vi "findcurrentpointinpath.vi"(9 "xyhc_in":T3={"idx"=1, "x"=-35.60561147, "y"=-90.69379038, "h"=0.8330275943157105, "x_path"=0.0}, 11 "path_updated":dbl[][](array[numeric])=[[-35.60561147, 14.99557688, 95.95172474, 126.8880385, 138.5119907, 141.9032354, 149.677826, 156.712601, 147.13884, 113.118729, 91.508095, 52.920765, 32.668774, 17.97715, 6.99827, 8.818146, 6.847322, -18.817772, -52.222027, -83.222168, -125.305626, -155.940872, -175.355911, -209.76741, -251.849823, -281.586182, -300.850311, -306.885162, -303.253143, -295.630493, -278.449524, -230.05719, -162.346695, -115.394356, -97.840988, -93.721558, -107.58947, -152.137314, -214.105331, -237.05452, -248.829102, -256.267426, -252.825378, -236.371918, -181.819519, -112.524597, -63.289055, 37.82652036, 102.9702202, 119.4941108, 132.2853204, 148.4183775, 169.4908835, 199.2599464, 217.8178611, 183.2960532, 161.2291024, 113.8171392, 51.7116428, 18.83330746, -40.94467646, -158.2175499, -304.1845662, -356.4114598, -371.7179639, -364.7774941, -321.8985356, -260.4948464, -177.352901, -134.2672684, -111.7310869, -102.4948394], [-90.69379038, -29.89498053, 67.16989543, 104.5939161, 124.5329647, 150.0144894, 165.817642, 203.642349, 245.81633, 291.834503, 311.325348, 320.550659, 312.945953, 299.664246, 267.743835, 241.541656, 208.411987, 171.587891, 162.666382, 167.037628, 157.857651, 138.040024, 134.616943, 139.73143, 136.464813, 119.024261, 90.540421, 58.270515, 37.237495, 23.16614, 14.112659, 28.614491, 56.741966, 65.419174, 53.848969, 35.074554, 14.354389, -0.839164, -11.569063, -18.164124, -25.487514, -39.475895, -50.265072, -60.782021, -86.859489, -89.836975, -52.336075, 47.42656259, 108.7608178, 124.5858933, 130.5720458, 134.255832, 156.1042719, 192.4121936, 263.2998005, 322.1206095, 338.63727, 360.3326326, 347.82789, 323.5375909, 277.8521386, 199.9919628, 130.779043, 91.89366581, 42.53528347, 5.307577259, -40.68181368, -69.83663356, -108.4425596, -125.3508342, -127.104311, -126.4810207], [0.8330275943157105, 0.8766933449672827, 0.8720608266883365, 0.8763291798774375, 1.4436202967580976, 1.0953588545336055, 1.202427103434421, 1.5675334075735572, 2.0208601993339705, 2.3344985584549347, 2.5217023998013075, 3.2905088869696257, 3.6946919524698116, 4.054443038499433, 4.694786404404647, 4.772122693546571, 4.485709108373563, 3.7189722485083774, 3.0712663600820562, 3.004853495888188, 3.7906498504911594, 3.507009551669314, 3.085443058474223, 3.0170500157627536, 3.451775038358818, 3.8955294400228175, 4.328504950817729, 4.7359268353628785, 5.031782879381744, 5.430482825844485, 6.2394321209923564, 6.667391813220487, 6.668706688268769, 6.092256265390278, 5.302149133586403, 4.529530775971869, 3.8056763953109787, 3.3266811332477855, 3.3420818347587327, 3.5361917912418064, 3.890153235193759, 4.650683955154467, 5.394163658376154, 5.775327394760227, 5.905741446161766, 6.685389788966887, 7.0624439921025415, 7.043797067523052, 7.045860587140642, 6.971258941777836, 6.421503011695177, 6.831190408876256, 7.153447806758524, 7.2239567423466955, 8.010347243061005, 8.72699497983693, 8.805052050684726, 9.26421305386915, 9.962792387892115, 10.087553564759371, 10.0731898733389, 9.920135612491762, 9.858317839615056, 10.401200892986212, 10.975024036193423, 11.393169003772442, 12.079383823703623, 12.12107561568999, 12.126125525723165, 12.365408786334852, 12.620725973569215, 12.60295968190307], [79.02567858668118, 126.39410707077633, 48.55371777691576, 22.760113207585164, 25.705859872710697, 17.609108944674627, 37.82045155891601, 42.14251814120699, 56.23518430452567, 29.023776728286606, 36.76726299353208, 21.15613435953993, 19.4783482417429, 31.97053018080938, 26.16608687203961, 32.95292667454974, 41.65012483034862, 32.85891459850081, 31.230672725830544, 40.43928661324237, 36.384170766299235, 19.35635780443436, 34.64429285631372, 41.35068505459292, 33.64069817064366, 33.54113151797454, 32.18140470915767, 21.112675843186466, 15.753153719369196, 18.122051452076935, 47.711722734111554, 73.31698058485364, 46.769151831896224, 19.43008535281352, 17.893999212117908, 22.89647093243486, 44.44498003577213, 62.884262384730775, 23.802898182097472, 13.685104750022273, 14.97011159822701, 10.556386662163115, 18.53445321010401, 60.34888944373504, 65.51457234068675, 59.98620700193982, 142.04554298999807, 89.47270858101754, 22.879495492192838, 13.682343682882424, 16.486885572353348, 29.369484986199453, 46.9472486010369, 68.21176822330133, 63.47923585020231, 27.521502278658343, 51.19605292655213, 59.307434583487634, 40.68066703288778, 75.23282019763789, 140.49305222582296, 161.32170793131496, 63.730285722300245, 49.46488273601802, 37.07722725836663, 59.00479817964879, 67.90876101874913, 91.66274958229026, 46.182949286236706, 22.432656547398086, 9.256469076869466, 11.245785601783329], [-6.993606016660986e-06, -1.5813147711021443e-07, -4.9412989479727785e-06, 0.0005804982640230092, -0.0005338958044692879, 0.00022896446877936018, 6.310818226633189e-06, 1.4800092263017844e-05, -1.6797654770616777e-05, 5.070149719265486e-05, 0.000115695865348633, 1.850562135420424e-06, 2.153681890354757e-05, 6.599016153961798e-05, -0.000141443646598775, -5.071687263203607e-05, -9.216151176499063e-05, -9.429046151669587e-05, 7.508132958046749e-05, 0.00016345906388144258, -0.00010687068557672743, -0.00016533777259995427, 9.565351143553687e-05, 3.201518460818227e-05, 2.438712115163615e-05, 9.20480250294573e-06, 2.72438887769066e-05, 1.734200726913153e-05, 0.00025540905209978505, 0.0008457169149239958, -0.0001053785279039084, -3.294439214038088e-06, -0.00010922182627835642, -0.00048481005659933374, -0.000594505792882455, -4.1701648383189044e-05, 9.000479999690469e-05, 1.0791978019384487e-05, 6.62890568708994e-05, 0.00022980729464205842, 0.0011537277543171918, 0.001279232309841406, -0.0007645391028542024, 1.953000206999253e-06, 6.836660316876013e-05, -3.111305584391926e-05, -8.652462043986586e-07, 1.5878703237004536e-06, -0.0001470721461860885, -0.0005412048195112028, 0.0009620023388559696, -0.00021848220595855873, 1.9545362257280654e-05, 4.665835242195117e-05, 2.1185462949283978e-05, -4.278663402683507e-05, 4.142252599915788e-05, 2.5234000269837195e-05, -4.337036628887736e-05, 1.0718640085458926e-06, -1.493391933607903e-06, 1.6667560305026813e-06, 4.541667742238345e-05, 1.6982539867374947e-05, 2.0938751238325963e-05, 2.3708700930883617e-05, -9.917110135809242e-06, -1.9179990515209864e-06, 5.213966173964119e-05, 2.6099096217165768e-05, -0.0005114331697200368, 0.002953773549767537], [0.0011054631256062924, 1.1654509850228165e-05, 0.000403832876154835, -0.005821160911709318, 0.013524571307922862, -0.0029959817275419303, 0.004695384990198625, 0.004844397614986437, 0.004300745221023324, 0.0010558943778921602, 0.006774386396445904, 0.010050228149390227, 0.009025536863599293, 0.008487959107981911, 0.007032289598104277, -0.0019617606126270115, -0.005807066954835113, -0.006865294004758757, -0.004582090071577949, 0.002458812820809224, 0.0018267420402203957, -0.0067836147414600916, -0.005959389502534751, 0.0036290335580481305, 0.005834877585639952, 0.006427345767029554, 0.005390142019435981, 0.006669244787197612, 0.007335460256323992, 0.005932688288565961, 0.012321999023593313, 0.00037127456573764255, 0.0007121496706068119, -0.01184694068062122, -0.011279978118629332, -0.017870097937325927, -0.011842834506194076, -0.0008955059357072287, 0.001762630905145975, 0.00878356216082013, 0.0058715751851772385, 0.023295289220100768, 0.032066762426306315, 0.0009098763678739921, 0.0008261134927424196, 0.006100298307186247, 0.00011871180816230411, -0.00020157501283942395, 0.0034140568922848727, -0.011285282284698564, -0.010620784317940626, 0.015309478200751929, -0.0006242166701697184, 0.002570702718513637, 0.004844470762756311, 0.0031873264917220956, 0.0016475340713924518, 0.004835739783382842, 0.004187930056684037, -0.00021642719823791983, -0.00023428081136886328, -0.0005951681406773184, 0.00039203631754227905, 0.005273623453740979, 0.004827688401290935, 0.004841657856736601, 0.0013173351453809295, 0.0002912599752114637, -0.0009707411088554158, 0.0049395054638412435, 0.0061413280612033026, -0.07414284312548818], [81.82977385474973, 130.0, 130.0, 21.51859834570865, 20.87556870416784, 34.01737307780925, 45.4310742849803, 43.292332385198996, 47.821782578933664, 43.98036931635985, 30.829418506724597, 32.09677212105701, 33.457332091579055, 32.04824819148381, 38.1954611577421, 40.65653867695928, 32.800429181663084, 31.915357946973696, 46.501222328543136, 30.098642621095763, 34.46178351366112, 28.727696585065573, 41.27703067679674, 41.939698880922464, 39.34171990650455, 39.52477756815426, 39.82632853043763, 38.28711226752185, 25.98064665063629, 19.52644932804886, 28.95642721008025, 130.0, 33.49359057360725, 21.61537706584067, 20.756214681085762, 23.776466260472024, 29.548817867613774, 80.94204546154333, 40.71960841866266, 26.12378716982201, 18.022289022120415, 16.331638316702904, 17.481096869630047, 78.72868682847616, 37.49106101741451, 40.832212096907085, 130.0, 130.0, 39.29804530301523, 21.19934187662583, 18.59438610567653, 25.87850238720156, 64.26226186149248, 40.111670137361685, 42.01051229834539, 54.3862369885448, 41.764322543788026, 41.255634426097615, 48.382793972933726, 130.0, 90.25544890626318, 100.9407983535582, 41.321049994965215, 41.73248472964462, 42.09739904900488, 41.53010736751869, 76.8285009124272, 130.0, 42.01973073534447, 40.94051358490329, 35.80543038271293, 11.860513000796347]]) -> (1 "xyhc_out":T3, 2 "xyhp":T2={"idx"=1, "x"=-33.26117542511643, "y"=-88.09498392627303, "hp"=0.8405086816068773, "x_path"=3.5})   [LabVIEW 2015]
uses:
  G_NAV.vi
  G_VEH.vi
  G_PATH.vi
panel:
  out "M6006":T1
  out "d0":dbl
  out "d1":dbl
  out "dm":dbl
  out "y-yv":dbl
  out "y-yv 2":dbl
  out "y-yv 3":dbl
  out "Path_c":dbl[](array[numeric]) format="%#_12g"
  out "x1":dbl format="%#_12g"
  out "xv":dbl format="%#_12g"
  out "yv":dbl format="%#_12g"
  out "x0":dbl format="%#_12g"
  out "xm":dbl
  out "path_idx_c":i32
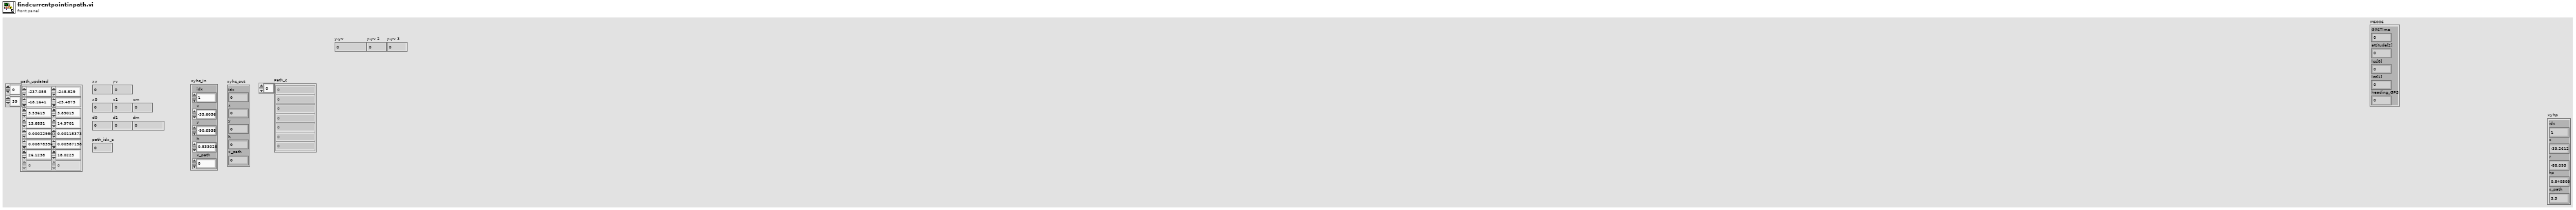
[diagram p1: front panel]
types:
  T1 = cluster{"GPSTime":dbl, "attitude[2]":sgl, "lcc[0]":sgl, "lcc[1]":sgl, "heading_GPS":sgl}
  T2 = cluster{"idx":i32, "x":dbl, "y":dbl, "hp":dbl, "x_path":dbl}
  T3 = cluster{"idx":i32, "x":dbl, "y":dbl, "h":dbl, "x_path":dbl}
  T4 = cluster{"Steer_input":dbl, "Steer_output":dbl, "VS_des":dbl, "VS_can":dbl, "heading":dbl, "auto":bool, "run":bool, "x":dbl, "y":dbl}
  T5 = cluster{"GPSTime":dbl, "attitude[2]":dbl, "lcc[0]":dbl, "lcc[1]":dbl, "heading_GPS":dbl}
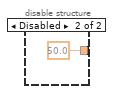
[diagram p3: hidden frame]
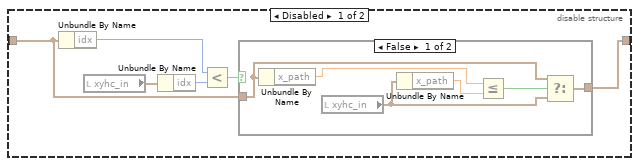
[diagram p6: hidden frame]
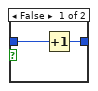
[diagram p9: hidden frame]
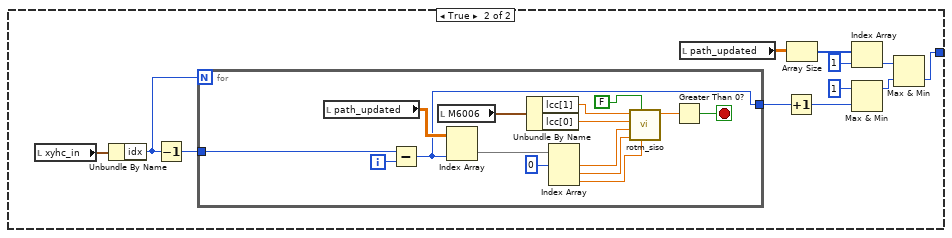
[diagram p10: hidden frame]
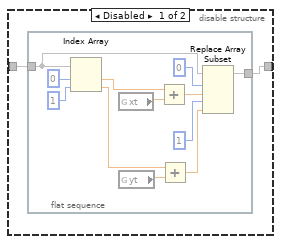
[diagram p11: hidden frame]
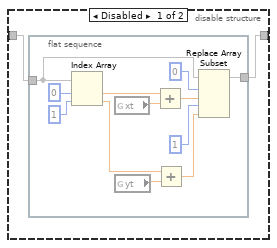
[diagram p12: hidden frame]
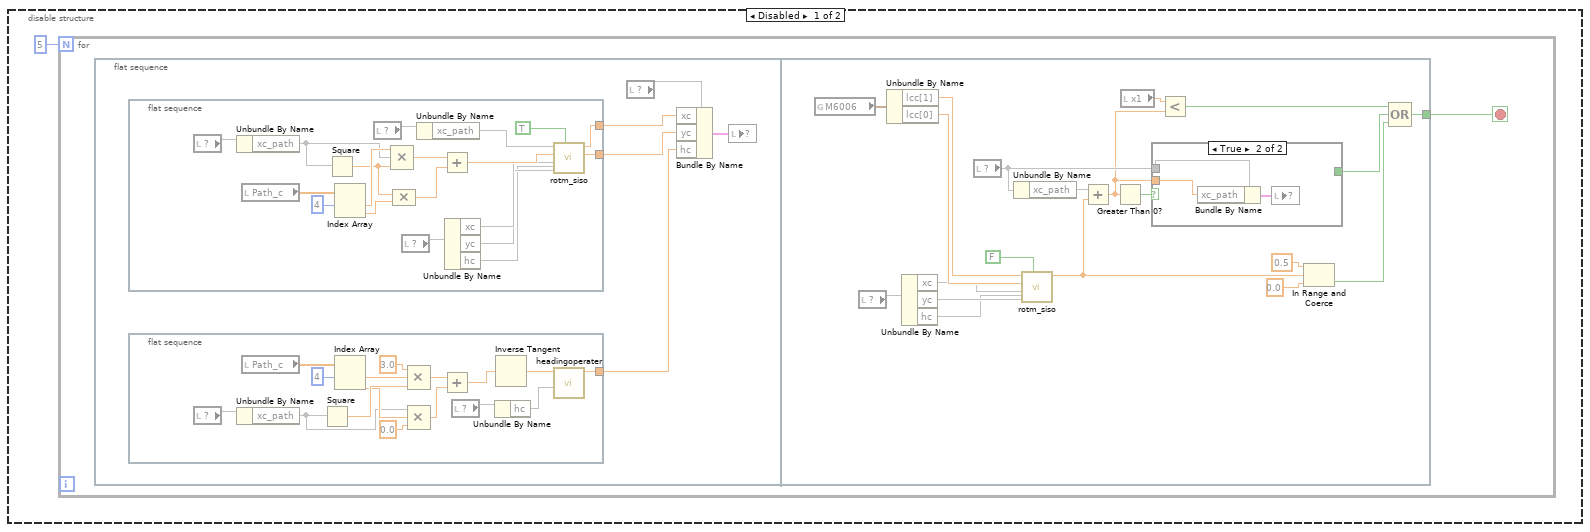
[diagram p15: hidden frame]
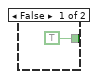
[diagram p16: hidden frame]
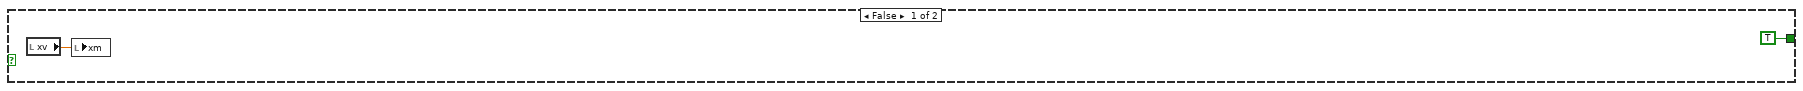
[diagram p17: hidden frame]
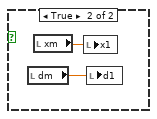
[diagram p19: hidden frame]
diagram:
  n1 = flat-sequence {
    frame #0 {
      n2 = disable-structure shown="Enabled" {
        disable-tunnel: [w21 50.0 ("Preview dist")] -> w9
        frame Enabled {
          n3 = global read "G_VEH.vi" "candata"() -> (w27:T4)
          n4 = Unbundle By Name(w27) -> ("VS_can"=w20:dbl)
          n5 = global read "G_VEH.vi" "preview_GAIN"() -> (w18:dbl)
          n6 = global read "G_VEH.vi" "max_preview"() -> (w25:dbl)
          n7 = global read "G_VEH.vi" "min_preview"() -> (w26:dbl)
          n8 = Divide(x=w20, y=3.6) -> (x/y=w19:dbl)
          n9 = Multiply(x=w19, y=w18) -> (x*y=w17:dbl)
          n10 = In Range and Coerce(upper limit=w25, x=w17, lower limit=w26) -> (coerced(x)=w22:dbl)  [unwired: 1 out]
          n11 = Add(x=w22, y=1.0) -> (x+y=w21:dbl)
        }
        frame Disabled {
        }
      }
      n12 = disable-structure shown="Disabled" {
        disable-tunnel: [w16 _] -> w8
        disable-tunnel: [w15 _] -> w3
        frame Disabled {
          n13 = global read "G_PATH.vi" "xt"() -> (w16:dbl)
          n14 = global read "G_PATH.vi" "yt"() -> (w15:dbl)
        }
        frame Enabled {
        }
      }
      n15 = global read "G_NAV.vi" "M6006"() -> (w7:T5)
      n16 = Unbundle By Name("xyhc_in") -> ("idx"=w14:i32)
      n17 = Unbundle By Name(w7) -> ("lcc[1]"=w6:dbl, "lcc[0]"=w4:dbl)
      n18 = Max & Min(x=w14, y=1) -> (max(x,y)=w13:i32)  [unwired: 1 out]
      n19 = Subtract(x=w6, y=w8) -> (x-y=w5:dbl)
      n20 = Subtract(x=w4, y=w3) -> (x-y=w2:dbl)
      n21 = Bundle By Name(cluster="xyhc_in", "idx"=w13) -> (w11:T3)
      n22 = local write "xyhc_in"(w11) -> ()
      n23 = Bundle By Name(cluster=w7, "lcc[1]"=w5, "lcc[0]"=w2) -> (→"M6006":T5)
      n24 = global write "G_VEH.vi" "Preview dist"(w9) -> ()
    }
    frame #1 {
      n25 = local read "path_updated"() -> (w34:dbl[][])
      n26 = Empty Array?(array=w34) -> (empty?=w35:bool)
      n27 = case shown="False" w35 {
        tunnel: [w70 T3 {"idx"=0, "x"=0.0, "y"=0.0, "h"=0.0, "x_path"=0.0} ("xyhc_out")] -> w30
        frame False {
          n28 = flat-sequence {
            tunnel: [w132] -> w69
            tunnel: w69 -> [w376]
            tunnel: [w425] -> w70
            frame #0 {
              n29 = global read "G_VEH.vi" "Reverse"() -> (w71:bool)
              n30 = case shown="False" w71 {
                tunnel: [w78 w110] -> w72
                frame False {
                  n31 = local read "path_updated"() -> (w86:dbl[][])
                  n32 = local read "xyhc_in"() -> (w76:T3)
                  n33 = Unbundle By Name(w76) -> ("idx"=w83:i32)
                  n34 = Array Size(array=w86) -> (size(s)=w85:i32[])
                  n35 = Decrement(x=w83) -> (x-1=w81:i32)
                  n36 = Index Array(array=w85, index=1) -> (element=w79:i32)
                  n37 = Subtract(x=w79, y=w81) -> (x-y=w82:i32)
                  n38 = for {
                    N: w82 -> [_]
                    tunnel: w81 -> [w103]
                    tunnel: [w94] -> w73
                    tunnel: [w93] -> w75
                    i -> [w104]
                    stop <- w93 stop-if-true
                    n39 = local read "path_updated"() -> (w102:dbl[][])
                    n40 = Add(x=w103, y=w104) -> (x+y=w94:i32)
                    n41 = local read "M6006"() -> (w90:T1)
                    n42 = Index Array(array=w102, index (col)=w94) -> (element=w97:dbl[])  [unwired: 1 in]
                    n43 = Unbundle By Name(w90) -> ("lcc[1]"=w99:sgl, "lcc[0]"=w98:sgl)
                    n44 = Index Array(array=w97, index #1=0 ("index")) -> (element #1=w92:dbl, element #2=w91:dbl, element #3=w100:dbl)  [unwired: 2 in]
                    n45 = call "rotm_siso.vi"("angle[rad]"=w100, "reverse"=FALSE, "y0"=w91, "x0"=w92, "y"=w98, "x"=w99) -> ("x'"=w95:dbl)  [unwired: 4 in, 1 out]
                    n46 = Less Than 0?(x=w95) -> (x < 0?=w93:bool)
                  }
                  n47 = case shown="True" w75 {
                    tunnel: [w87 w89] -> w74
                    tunnel: w73 -> [w88 w89]
                    frame False {
                      n48 = Increment(x=w88) -> (x+1=w87:i32)
                    }
                    frame True {
                    }
                  }
                  n49 = Max & Min(x=1, y=w74) -> (max(x,y)=w77:i32)  [unwired: 1 out]
                  n50 = Max & Min(x=w79, y=w77) -> (min(x,y)=w78:i32)  [unwired: 1 out]
                }
                frame True {
                  n51 = local read "xyhc_in"() -> (w108:T3)
                  n52 = Unbundle By Name(w108) -> ("idx"=w107:i32)
                  n53 = Decrement(x=w107) -> (x-1=w113:i32)
                  n54 = for {
                    N: w107 -> [_]
                    tunnel: w113 -> [w130]
                    tunnel: [w118] -> w106
                    i -> [w131]
                    stop <- w119 stop-if-true
                    n55 = local read "path_updated"() -> (w129:dbl[][])
                    n56 = Subtract(x=w130, y=w131) -> (x-y=w118:i32)
                    n57 = local read "M6006"() -> (w117:T1)
                    n58 = Index Array(array=w129, index (col)=w118) -> (element=w122:dbl[])  [unwired: 1 in]
                    n59 = Unbundle By Name(w117) -> ("lcc[1]"=w124:sgl, "lcc[0]"=w123:sgl)
                    n60 = Index Array(array=w122, index #1=0 ("index")) -> (element #1=w127:dbl, element #2=w126:dbl, element #3=w125:dbl)  [unwired: 2 in]
                    n61 = call "rotm_siso.vi"("angle[rad]"=w125, "reverse"=FALSE, "y0"=w126, "x0"=w127, "y"=w123, "x"=w124) -> ("x'"=w120:dbl)  [unwired: 4 in, 1 out]
                    n62 = Greater Than 0?(x=w120) -> (x > 0?=w119:bool)
                  }
                  n63 = local read "path_updated"() -> (w116:dbl[][])
                  n64 = Increment(x=w106) -> (x+1=w105:i32)
                  n65 = Array Size(array=w116) -> (size(s)=w115:i32[])
                  n66 = Index Array(array=w115, index=1) -> (element=w111:i32)
                  n67 = Max & Min(x=1, y=w105) -> (max(x,y)=w109:i32)  [unwired: 1 out]
                  n68 = Max & Min(x=w111, y=w109) -> (min(x,y)=w110:i32)  [unwired: 1 out]
                }
              }
              "path_idx_c" <- w72
            }
            frame #1 {
              n69 = flat-sequence {
                tunnel: [w267] -> w132
                frame #0 {
                  w139 = 0.0 ("y")
                  n70 = local read "path_idx_c"() -> (w141:i32)
                  n71 = local read "path_updated"() -> (w147:dbl[][])
                  n72 = Decrement(x=w141) -> (x-1=w153:i32)
                  n73 = Index Array(array=w147, index (col)=w153) -> (element=w137:dbl[])  [unwired: 1 in]
                  n74 = disable-structure shown="Enabled" {
                    disable-tunnel: w137 -> [w155 w168]
                    disable-tunnel: [w154 w168] -> w136
                    frame Disabled {
                      n75 = flat-sequence {
                        tunnel: w155 -> [w165]
                        tunnel: [w164] -> w154
                        frame #0 {
                          n76 = Index Array(array=w165, index #1=0 ("index"), index #2=1 ("index")) -> (element #1=w162:dbl, element #2=w159:dbl)
                          n77 = global read "G_PATH.vi" "xt"() -> (w167:dbl)
                          n78 = global read "G_PATH.vi" "yt"() -> (w166:dbl)
                          n79 = Add(x=w162, y=w167) -> (x+y=w160:dbl)
                          n80 = Add(x=w159, y=w166) -> (x+y=w158:dbl)
                          n81 = Replace Array Subset(array=w165, new element #1=w160, index #1=0 ("index"), new element #2=w158, index #2=1 ("index")) -> (w164:dbl[])
                        }
                      }
                    }
                    frame Enabled {
                    }
                  }
                  "Path_c" <- w136
                  n82 = local read "M6006"() -> (w133:T1)
                  n83 = Unbundle By Name(w133) -> ("lcc[1]"=w152:sgl, "lcc[0]"=w151:sgl)
                  n84 = Index Array(array=w136, index #1=3 ("index"), index #2=0 ("index")) -> (element #1=w138:dbl, element #2=w135:dbl, element #3=w134:dbl, element #4=w148:dbl)  [unwired: 3 in, 1 out]
                  "x1" <- w138
                  n85 = Add(x=w139, y=w138) -> (x+y=w145:dbl)
                  n86 = call "rotm_siso.vi"("angle[rad]"=w148, "reverse"=FALSE, "y0"=w134, "x0"=w135, "y"=w151, "x"=w152) -> ("y'"=→"yv":dbl, "x'"=→"xv":dbl)  [unwired: 4 in]
                  n87 = Multiply(x=w145, y=0.5) -> (x*y=→"xm":dbl)
                  "x0" <- w139
                }
                frame #1 {
                  n88 = local read "Path_c"() -> (w195:dbl[])
                  n89 = local read "Path_c"() -> (w179:dbl[])
                  n90 = local read "Path_c"() -> (w180:dbl[])
                  n91 = Index Array(array=w195, index #1=4 ("index")) -> (element #1=w193:dbl, element #2=w192:dbl)  [unwired: 1 in]
                  n92 = Index Array(array=w179, index #1=4 ("index")) -> (element #1=w177:dbl, element #2=w176:dbl)  [unwired: 1 in]
                  n93 = Index Array(array=w180, index #1=4 ("index")) -> (element #1=w182:dbl, element #2=w183:dbl)  [unwired: 1 in]
                  n94 = local read "x0"() -> (w191:dbl)
                  n95 = local read "xv"() -> (w190:dbl)
                  n96 = local read "yv"() -> (w189:dbl)
                  n97 = local read "xm"() -> (w172:dbl)
                  n98 = local read "xv"() -> (w175:dbl)
                  n99 = local read "yv"() -> (w174:dbl)
                  n100 = local read "x1"() -> (w184:dbl)
                  n101 = local read "xv"() -> (w185:dbl)
                  n102 = local read "yv"() -> (w186:dbl)
                  n103 = call "distfc.vi"("a"=w193, "b"=w192, "x"=w191, "xv"=w190, "yv"=w189) -> ("d"=→"d0":dbl, "y-yv"=→"y-yv":dbl)  [unwired: 9 in]
                  n104 = call "distfc.vi"("a"=w182, "b"=w183, "x"=w184, "xv"=w185, "yv"=w186) -> ("d"=→"d1":dbl, "y-yv"=→"y-yv 2":dbl)  [unwired: 9 in]
                  n105 = call "distfc.vi"("a"=w177, "b"=w176, "x"=w172, "xv"=w175, "yv"=w174) -> ("d"=→"dm":dbl, "y-yv"=→"y-yv 3":dbl)  [unwired: 9 in]
                }
                frame #2 {
                  n106 = local read "xv"() -> (w197:dbl)
                  n107 = local read "x1"() -> (w198:dbl)
                  n108 = Less Or Equal?(x=w197, y=w198) -> (x <= y?=w196:bool)
                  n109 = case shown="False" w196 {
                    frame False {
                      n110 = local read "path_updated"() -> (w202:dbl[][])
                      n111 = local read "path_idx_c"() -> (w201:i32)
                      n112 = Index Array(array=w202, index (col)=w201) -> (element=w199:dbl[])  [unwired: 1 in]
                      n113 = Empty Array?(array=w199) -> (empty?=w200:bool)
                      n114 = case shown="False" w200 {
                        tunnel: w199 -> [w204 _]
                        frame False {
                          n115 = flat-sequence {
                            tunnel: w204 -> [w206]
                            tunnel: [w205] -> w203
                            tunnel: w203 -> [w230]
                            frame #0 {
                              n116 = disable-structure shown="Enabled" {
                                disable-tunnel: w206 -> [w208 w221]
                                disable-tunnel: [w207 w221] -> w205
                                frame Disabled {
                                n117 = flat-sequence {
                                tunnel: w208 -> [w218]
                                tunnel: [w217] -> w207
                                frame #0 {
                                n118 = Index Array(array=w218, index #1=0 ("index"), index #2=1 ("index")) -> (element #1=w215:dbl, element #2=w212:dbl)
                                n119 = global read "G_PATH.vi" "xt"() -> (w220:dbl)
                                n120 = global read "G_PATH.vi" "yt"() -> (w219:dbl)
                                n121 = Add(x=w215, y=w220) -> (x+y=w213:dbl)
                                n122 = Add(x=w212, y=w219) -> (x+y=w211:dbl)
                                n123 = Replace Array Subset(array=w218, new element #1=w213, index #1=0 ("index"), new element #2=w211, index #2=1 ("index")) -> (w217:dbl[])
                                }
                                }
                                }
                                frame Enabled {
                                }
                              }
                            }
                            frame #1 {
                              w228 = 0.0 ("y")
                              n124 = local write "Path_c"(w230) -> ()
                              n125 = local read "M6006"() -> (w222:T1)
                              n126 = local read "path_idx_c"() -> (w224:i32)
                              n127 = Unbundle By Name(w222) -> ("lcc[1]"=w231:sgl, "lcc[0]"=w232:sgl)
                              n128 = Index Array(array=w230, index #1=0 ("index")) -> (element #1=w235:dbl, element #2=w236:dbl, element #3=w237:dbl, element #4=w229:dbl)  [unwired: 3 in]
                              n129 = local write "x0"(w228) -> ()
                              n130 = local write "x1"(w229) -> ()
                              n131 = Increment(x=w224) -> (x+1=w223:i32)
                              n132 = Add(x=w229, y=w228) -> (x+y=w238:dbl)
                              n133 = local write "path_idx_c"(w223) -> ()
                              n134 = call "rotm_siso.vi"("angle[rad]"=w237, "reverse"=FALSE, "y0"=w236, "x0"=w235, "y"=w232, "x"=w231) -> ("y'"=w225:dbl, "x'"=w226:dbl)  [unwired: 4 in]
                              n135 = local write "xv"(w226) -> ()
                              n136 = local write "yv"(w225) -> ()
                              n137 = Multiply(x=w238, y=0.5) -> (x*y=w227:dbl)
                              n138 = local write "xm"(w227) -> ()
                            }
                            frame #2 {
                              n139 = local read "Path_c"() -> (w246:dbl[])
                              n140 = local read "Path_c"() -> (w260:dbl[])
                              n141 = local read "Path_c"() -> (w259:dbl[])
                              n142 = Index Array(array=w246, index #1=4 ("index")) -> (element #1=w248:dbl, element #2=w249:dbl)  [unwired: 3 in, 2 out]
                              n143 = Index Array(array=w260, index #1=4 ("index")) -> (element #1=w262:dbl, element #2=w263:dbl)  [unwired: 3 in, 2 out]
                              n144 = Index Array(array=w259, index #1=4 ("index")) -> (element #1=w257:dbl, element #2=w256:dbl)  [unwired: 3 in, 2 out]
                              n145 = local read "x0"() -> (w250:dbl)
                              n146 = local read "xv"() -> (w251:dbl)
                              n147 = local read "yv"() -> (w252:dbl)
                              n148 = local read "xm"() -> (w266:dbl)
                              n149 = local read "xv"() -> (w264:dbl)
                              n150 = local read "yv"() -> (w265:dbl)
                              n151 = local read "x1"() -> (w255:dbl)
                              n152 = local read "xv"() -> (w254:dbl)
                              n153 = local read "yv"() -> (w253:dbl)
                              n154 = call "distfc.vi"("a"=w248, "b"=w249, "x"=w250, "xv"=w251, "yv"=w252) -> ("d"=w243:dbl, "y-yv"=w242:dbl)  [unwired: 9 in]
                              n155 = call "distfc.vi"("a"=w257, "b"=w256, "x"=w255, "xv"=w254, "yv"=w253) -> ("d"=w241:dbl, "y-yv"=w240:dbl)  [unwired: 9 in]
                              n156 = call "distfc.vi"("a"=w262, "b"=w263, "x"=w266, "xv"=w264, "yv"=w265) -> ("d"=w245:dbl, "y-yv"=w244:dbl)  [unwired: 9 in]
                              n157 = local write "d0"(w243) -> ()
                              n158 = local write "y-yv"(w242) -> ()
                              n159 = local write "dm"(w245) -> ()
                              n160 = local write "y-yv 3"(w244) -> ()
                              n161 = local write "d1"(w241) -> ()
                              n162 = local write "y-yv 2"(w240) -> ()
                            }
                          }
                        }
                        frame True {
                        }
                      }
                    }
                    frame True {
                    }
                  }
                }
                frame #3 {
                  n163 = disable-structure shown="Enabled" {
                    disable-tunnel: [_ w334] -> w267
                    frame Disabled {
                      n164 = for {
                        N: 5 -> [_]
                        stop <- w269 stop-if-true
                        n165 = flat-sequence {
                          tunnel: [w313] -> w269
                          frame #0 {
                            n166 = flat-sequence {
                              tunnel: [w292] -> w274
                              tunnel: [w291] -> w273
                              frame #0 {
                                n167 = local read item#-1() -> (w300)
                                n168 = Unbundle By Name(w300) -> ("xc_path"=w299)
                                n169 = local read "Path_c"() -> (w303:dbl[])
                                n170 = Square(x=w299) -> (x^2=w304:dbl)
                                n171 = Index Array(array=w303, index #1=4 ("index")) -> (element #1=w308:dbl, element #2=w307:dbl)  [unwired: 1 in]
                                n172 = local read item#-1() -> (w298)
                                n173 = Compound Arithmetic op=MULTIPLY(w308, w299, w304) -> (w306:dbl)
                                n174 = Compound Arithmetic op=MULTIPLY(w304, w307) -> (w305:dbl)
                                n175 = local read item#-1() -> (w296)
                                n176 = Unbundle By Name(w298) -> ("xc_path"=w297)
                                n177 = Add(x=w306, y=w305) -> (x+y=w302:dbl)
                                n178 = Unbundle By Name(w296) -> ("xc"=w295, "yc"=w294, "hc"=w293)
                                n179 = call "rotm_siso.vi"("angle[rad]"=w293, "reverse"=TRUE, "y0"=w294, "x0"=w295, "y"=w302, "x"=w297) -> ("y'"=w291:dbl, "x'"=w292:dbl)  [unwired: 4 in]
                              }
                            }
                            n180 = flat-sequence {
                              tunnel: [w275] -> w271
                              frame #0 {
                                n181 = local read item#-1() -> (w290)
                                n182 = Unbundle By Name(w290) -> ("xc_path"=w282)
                                n183 = local read "Path_c"() -> (w289:dbl[])
                                n184 = Square(x=w282) -> (x^2=w285:dbl)
                                n185 = Index Array(array=w289, index #1=4 ("index")) -> (element #1=w287:dbl, element #2=w284:dbl)  [unwired: 1 in]
                                n186 = Compound Arithmetic op=MULTIPLY(3.0 ("value"), w287, w285) -> (w281:dbl)
                                n187 = Compound Arithmetic op=MULTIPLY(w282, w284, 0.0 ("value")) -> (w280:dbl)
                                n188 = Add(x=w281, y=w280) -> (x+y=w279:dbl)
                                n189 = local read item#-1() -> (w278)
                                n190 = Unbundle By Name(w278) -> ("hc"=w276)
                                n191 = Inverse Tangent(1:w279) -> (0:w277:dbl)
                                n192 = call "headingoperater.vi"("h1"=w276, "h2"=w277) -> ("h2+h1"=w275:dbl)  [unwired: 8 in, 1 out]
                              }
                            }
                            n193 = local read item#-1() -> (w272)
                            n194 = Bundle By Name(cluster=w272, "xc"=w274, "yc"=w273, "hc"=w271) -> (w270:cluster{})
                            n195 = local write item#-1(w270) -> ()
                          }
                          frame #1 {
                            n196 = global read "G_NAV.vi" "M6006"() -> (w326:T5)
                            n197 = local read item#-1() -> (w325)
                            n198 = Unbundle By Name(w326) -> ("lcc[1]"=w327:dbl, "lcc[0]"=w328:dbl)
                            n199 = Unbundle By Name(w325) -> ("xc"=w324, "yc"=w323, "hc"=w322)
                            n200 = local read item#-1() -> (w321)
                            n201 = Unbundle By Name(w321) -> ("xc_path"=w320)
                            n202 = call "rotm_siso.vi"("angle[rad]"=w322, "reverse"=FALSE, "y0"=w323, "x0"=w324, "y"=w328, "x"=w327) -> ("x'"=w317:dbl)  [unwired: 4 in, 1 out]
                            n203 = Add(x=w320, y=w317) -> (x+y=w311:dbl)
                            n204 = Greater Than 0?(x=w311) -> (x > 0?=w316:bool)
                            n205 = local read "x1"() -> (w312:dbl)
                            n206 = case shown="True" w316 {
                              tunnel: w321 -> [_ w332]
                              tunnel: w311 -> [_ w331]
                              tunnel: [TRUE _] -> w315
                              frame False {
                              }
                              frame True {
                                n207 = Bundle By Name(cluster=w332, "xc_path"=w331) -> (w333:cluster{})
                                n208 = local write item#-1(w333) -> ()
                              }
                            }
                            n209 = Less?(x=w312, y=w311) -> (x < y?=w310:bool)
                            n210 = In Range and Coerce(upper limit=0.5, x=w317, lower limit=0.0) -> (In Range?=w314:bool)  [unwired: 1 out]
                            n211 = Compound Arithmetic op=OR(w310, w315, w314) -> (w313:bool)
                          }
                        }
                      }
                    }
                    frame Enabled {
                      n212 = local read "xv"() -> (w340:dbl)
                      n213 = local read "xv"() -> (w339:dbl)
                      n214 = local read "x1"() -> (w338:dbl)
                      n215 = Greater Than 0?(x=w340) -> (x > 0?=w337:bool)
                      n216 = Less Or Equal?(x=w339, y=w338) -> (x <= y?=w336:bool)
                      n217 = And(x=w337, y=w336) -> (x .and. y?=w335:bool)
                      n218 = case shown="True" w335 {
                        tunnel: [TRUE w343] -> w334
                        frame False {
                          n219 = local read "xv"() -> (w342:dbl)
                          n220 = local write "xm"(w342) -> ()
                        }
                        frame True {
                          n221 = for {
                            N: 20 -> [_]
                            tunnel: [w345] -> w343
                            stop <- w345 stop-if-true
                            n222 = flat-sequence {
                              tunnel: [w365] -> w345
                              frame #0 {
                                n223 = local read "dm"() -> (w349:dbl)
                                n224 = local read "d0"() -> (w350:dbl)
                                n225 = Multiply(x=w350, y=w349) -> (x*y=w348:dbl)
                                n226 = Sign(1:w348) -> (0:w347:dbl)
                                n227 = Less Or Equal To 0?(x=w347) -> (x <= 0?=w346:bool)
                                n228 = case shown="False" w346 {
                                frame False {
                                n229 = local read "dm"() -> (w354:dbl)
                                n230 = local read "d1"() -> (w355:dbl)
                                n231 = Multiply(x=w355, y=w354) -> (x*y=w353:dbl)
                                n232 = Sign(1:w353) -> (0:w352:dbl)
                                n233 = Less Or Equal To 0?(x=w352) -> (x <= 0?=w351:bool)
                                n234 = case shown="True" w351 {
                                frame False {
                                }
                                frame True {
                                n235 = local read "dm"() -> (w356:dbl)
                                n236 = local read "xm"() -> (w357:dbl)
                                n237 = local write "x0"(w357) -> ()
                                n238 = local write "d0"(w356) -> ()
                                }
                                }
                                }
                                frame True {
                                n239 = local read "dm"() -> (w358:dbl)
                                n240 = local read "xm"() -> (w359:dbl)
                                n241 = local write "x1"(w359) -> ()
                                n242 = local write "d1"(w358) -> ()
                                }
                                }
                              }
                              frame #1 {
                                n243 = local read "x0"() -> (w364:dbl)
                                n244 = local read "x1"() -> (w363:dbl)
                                n245 = Add(x=w364, y=w363) -> (x+y=w362:dbl)
                                n246 = Multiply(x=w362, y=0.5) -> (x*y=w360:dbl)
                                n247 = local write "xm"(w360) -> ()
                              }
                              frame #2 {
                                n248 = local read "Path_c"() -> (w375:dbl[])
                                n249 = Index Array(array=w375, index #1=4 ("index")) -> (element #1=w373:dbl, element #2=w372:dbl)  [unwired: 1 in]
                                n250 = local read "xm"() -> (w369:dbl)
                                n251 = local read "xv"() -> (w371:dbl)
                                n252 = local read "yv"() -> (w370:dbl)
                                n253 = call "distfc.vi"("a"=w373, "b"=w372, "x"=w369, "xv"=w371, "yv"=w370) -> ("d"=w368:dbl)  [unwired: 9 in, 1 out]
                                n254 = local write "dm"(w368) -> ()
                                n255 = Absolute Value(x=w368) -> (abs(x)=w367:dbl)
                                n256 = Less?(x=w367, y=0.001) -> (x < y?=w365:bool)
                              }
                            }
                          }
                        }
                      }
                    }
                  }
                }
              }
            }
            frame #2 {
              n257 = case shown="False" w376 {
                frame False {
                  n258 = local read "Path_c"() -> (w390:dbl[])
                  n259 = local read "Path_c"() -> (w404:dbl[])
                  n260 = local read "Path_c"() -> (w403:dbl[])
                  n261 = local read "Path_c"() -> (w411:dbl[])
                  n262 = Index Array(array=w390, index #1=4 ("index")) -> (element #1=w392:dbl, element #2=w393:dbl)  [unwired: 1 in]
                  n263 = Index Array(array=w404, index #1=4 ("index")) -> (element #1=w406:dbl, element #2=w407:dbl)  [unwired: 1 in]
                  n264 = Index Array(array=w403, index #1=4 ("index")) -> (element #1=w401:dbl, element #2=w400:dbl)  [unwired: 1 in]
                  n265 = Index Array(array=w411, index #1=4 ("index")) -> (element #1=w413:dbl, element #2=w414:dbl)  [unwired: 1 in]
                  n266 = local read "x0"() -> (w394:dbl)
                  n267 = local read "xv"() -> (w395:dbl)
                  n268 = local read "yv"() -> (w396:dbl)
                  n269 = local read "xm"() -> (w410:dbl)
                  n270 = local read "xv"() -> (w408:dbl)
                  n271 = local read "yv"() -> (w409:dbl)
                  n272 = local read "x1"() -> (w399:dbl)
                  n273 = local read "xv"() -> (w398:dbl)
                  n274 = local read "yv"() -> (w397:dbl)
                  n275 = local read "xv"() -> (w417:dbl)
                  n276 = local read "xv"() -> (w415:dbl)
                  n277 = local read "yv"() -> (w416:dbl)
                  n278 = call "distfc.vi"("a"=w392, "b"=w393, "x"=w394, "xv"=w395, "yv"=w396) -> ("d"=w389:dbl)  [unwired: 9 in, 1 out]
                  n279 = call "distfc.vi"("a"=w401, "b"=w400, "x"=w399, "xv"=w398, "yv"=w397) -> ("d"=w387:dbl)  [unwired: 9 in, 1 out]
                  n280 = call "distfc.vi"("a"=w413, "b"=w414, "x"=w417, "xv"=w415, "yv"=w416) -> ("d"=w386:dbl)  [unwired: 9 in, 1 out]
                  n281 = call "distfc.vi"("a"=w406, "b"=w407, "x"=w410, "xv"=w408, "yv"=w409) -> ("d"=w388:dbl)  [unwired: 9 in, 1 out]
                  n282 = Build Array(w389, w388, w387, w386) -> (w385:dbl[])
                  n283 = Absolute Value(x=w385) -> (abs(x)=w384:dbl[])
                  n284 = local read "x0"() -> (w383:dbl)
                  n285 = local read "xm"() -> (w382:dbl)
                  n286 = local read "x1"() -> (w381:dbl)
                  n287 = local read "xv"() -> (w380:dbl)
                  n288 = Array Max & Min(array=w384) -> (min index (indices)=w378:i32)  [unwired: 3 out]
                  n289 = Build Array(w383, w382, w381, w380) -> (w379:dbl[])
                  n290 = Index Array(array=w379, index=w378) -> (element=w377:dbl)
                  n291 = local write "xm"(w377) -> ()
                }
                frame True {
                }
              }
            }
            frame #3 {
              n292 = local read "path_idx_c"() -> (w427:i32)
              n293 = local read "path_updated"() -> (w428:dbl[][])
              n294 = Decrement(x=w427) -> (x-1=w451:i32)
              n295 = Index Array(array=w428, index (col)=w451) -> (element=w419:dbl[])  [unwired: 1 in]
              n296 = disable-structure shown="Enabled" {
                disable-tunnel: w419 -> [w457 w470]
                disable-tunnel: [w456 w470] -> w418
                frame Disabled {
                  n297 = flat-sequence {
                    tunnel: w457 -> [w467]
                    tunnel: [w466] -> w456
                    frame #0 {
                      n298 = Index Array(array=w467, index #1=0 ("index"), index #2=1 ("index")) -> (element #1=w464:dbl, element #2=w461:dbl)
                      n299 = global read "G_PATH.vi" "xt"() -> (w469:dbl)
                      n300 = global read "G_PATH.vi" "yt"() -> (w468:dbl)
                      n301 = Add(x=w464, y=w469) -> (x+y=w462:dbl)
                      n302 = Add(x=w461, y=w468) -> (x+y=w460:dbl)
                      n303 = Replace Array Subset(array=w467, new element #1=w462, index #1=0 ("index"), new element #2=w460, index #2=1 ("index")) -> (w466:dbl[])
                    }
                  }
                }
                frame Enabled {
                }
              }
              n304 = local read "xm"() -> (w424:dbl)
              n305 = local read "xm"() -> (w423:dbl)
              n306 = Index Array(array=w418, index #1=5 ("index"), index #2=4 ("index"), index #3=0 ("index"), index #6=4 ("index")) -> (element #1=w432:dbl, element #2=w453:dbl, element #3=w447:dbl, element #4=w446:dbl, element #5=w431:dbl, element #6=w440:dbl, element #7=w438:dbl)  [unwired: 3 in]
              n307 = Square(x=w424) -> (x^2=w452:dbl)
              n308 = Square(x=w423) -> (x^2=w439:dbl)
              n309 = Compound Arithmetic op=MULTIPLY(w452, w424, w453) -> (w455:dbl)
              n310 = Compound Arithmetic op=MULTIPLY(w432, w452) -> (w454:dbl)
              n311 = Compound Arithmetic op=MULTIPLY(3.0 ("value"), w440, w439) -> (w437:dbl)
              n312 = Compound Arithmetic op=MULTIPLY(w423, w438, 2.0 ("value")) -> (w436:dbl)
              n313 = Add(x=w454, y=w455) -> (x+y=w449:dbl)
              n314 = Add(x=w437, y=w436) -> (x+y=w435:dbl)
              n315 = local read "xm"() -> (w421:dbl)
              n316 = Inverse Tangent(1:w435) -> (0:w430:dbl)
              n317 = local read "path_idx_c"() -> (w426:i32)
              n318 = call "rotm_siso.vi"("angle[rad]"=w431, "reverse"=TRUE, "y0"=w446, "x0"=w447, "y"=w449, "x"=w421) -> ("y'"=w444:dbl, "x'"=w445:dbl)  [unwired: 4 in]
              n319 = call "headingoperater.vi"("h1"=w430, "h2"=w431) -> ("h2+h1"=w429:dbl)  [unwired: 8 in, 1 out]
              n320 = local read "xm"() -> (w422:dbl)
              n321 = Bundle By Name(cluster=T3 {"idx"=0, "x"=0.0, "y"=0.0, "h"=0.0, "x_path"=0.0} ("xyhc_out"), "idx"=w426, "x"=w445, "y"=w444, "h"=w429, "x_path"=w422) -> (w425:T3)
            }
          }
        }
        frame True {
        }
      }
      n322 = global read "G_VEH.vi" "candata"() -> (w33:T4)
      n323 = Unbundle By Name(w33) -> ("VS_can"=w32:dbl)
      n324 = Greater Or Equal To 0?(x=w32) -> (x >= 0?=w31:bool)
      n325 = disable-structure shown="Enabled" {
        disable-tunnel: w31 -> [w38 _]
        disable-tunnel: w30 -> [w37 w68]
        disable-tunnel: [w36 w68] -> w29
        frame Enabled {
          n326 = case shown="True" w38 {
            tunnel: w37 -> [w43 w52]
            tunnel: [w44 w53] -> w36
            frame True {
              n327 = Unbundle By Name(w43) -> ("idx"=w41:i32)
              n328 = local read "xyhc_in"() -> (w42:T3)
              n329 = Unbundle By Name(w42) -> ("idx"=w40:i32)
              n330 = Greater?(x=w41, y=w40) -> (0:w39:bool)
              n331 = case shown="False" w39 {
                tunnel: [w45 w51] -> w44
                tunnel: w43 -> [w47 w51]
                frame False {
                  n332 = Unbundle By Name(w47) -> ("x_path"=w49:dbl)
                  n333 = local read "xyhc_in"() -> (w46:T3)
                  n334 = Unbundle By Name(w46) -> ("x_path"=w50:dbl)
                  n335 = Greater Or Equal?(x=w49, y=w50) -> (x >= y?=w48:bool)
                  n336 = Select(t=w47, s=w48, f=w46) -> (s? t:f=w45:T3)
                }
                frame True {
                }
              }
            }
            frame False {
              n337 = disable-structure shown="Enabled" {
                disable-tunnel: [w55 w67] -> w53
                disable-tunnel: w52 -> [w54 w67]
                frame Disabled {
                  n338 = Unbundle By Name(w54) -> ("idx"=w58:i32)
                  n339 = local read "xyhc_in"() -> (w59:T3)
                  n340 = Unbundle By Name(w59) -> ("idx"=w57:i32)
                  n341 = Less?(x=w58, y=w57) -> (x < y?=w56:bool)
                  n342 = case shown="False" w56 {
                    tunnel: [w60 w66] -> w55
                    tunnel: w54 -> [w62 w66]
                    frame False {
                      n343 = Unbundle By Name(w62) -> ("x_path"=w64:dbl)
                      n344 = local read "xyhc_in"() -> (w61:T3)
                      n345 = Unbundle By Name(w61) -> ("x_path"=w65:dbl)
                      n346 = Less Or Equal?(x=w64, y=w65) -> (x <= y?=w63:bool)
                      n347 = Select(t=w62, s=w63, f=w61) -> (s? t:f=w60:T3)
                    }
                    frame True {
                    }
                  }
                }
                frame Enabled {
                }
              }
            }
          }
        }
        frame Disabled {
        }
      }
      "xyhc_out" <- w29
    }
    frame #2 {
      n348 = local read "path_updated"() -> (w473:dbl[][])
      n349 = Empty Array?(array=w473) -> (empty?=w474:bool)
      n350 = case shown="False" w474 {
        tunnel: [w475 T2 {"idx"=0, "x"=0.0, "y"=0.0, "hp"=0.0, "x_path"=0.0} ("xyhp")] -> w472
        frame False {
          n351 = local read "xyhc_out"() -> (w487:T3)
          n352 = local read "path_updated"() -> (w490:dbl[][])
          n353 = local read "xyhc_out"() -> (w483:T3)
          n354 = Unbundle By Name(w487) -> ("idx"=w480:i32)
          n355 = global read "G_VEH.vi" "Preview dist"() -> (w482:dbl)
          n356 = Unbundle By Name(w483) -> ("x_path"=w481:dbl)
          n357 = Decrement(x=w480) -> (x-1=w486:i32)
          n358 = Index Array(array=w490, index (row)=3) -> (element=w488:dbl[])  [unwired: 1 in]
          n359 = Add(x=w482, y=w481) -> (x+y=w479:dbl)
          n360 = Split 1D Array(array=w488, index=w486) -> (second subarray=w485:dbl[])  [unwired: 1 out]
          n361 = for {
            tunnel: w485 -> [w555] mode=indexing
            shift-right: [w554] -> _
            shift-left: 0.0 -> [w553]
            tunnel: w479 -> [w552]
            tunnel: [w551] -> w478
            tunnel: [w550] -> w477
            tunnel: [w549] -> w476
            i -> [w549]
            stop <- w550 stop-if-true
            n362 = Subtract(x=w552, y=w553) -> (x-y=w551:dbl)
            n363 = Add(x=w553, y=w555) -> (x+y=w554:dbl)
            n364 = Greater?(x=w554, y=w552) -> (0:w550:bool)
          }
          n365 = case shown="True" w477 {
            tunnel: w478 -> [_ w499]
            tunnel: w476 -> [_ w497]
            tunnel: [T2 {"idx"=0, "x"=0.0, "y"=0.0, "hp"=0.0, "x_path"=0.0} ("xyhp") w495] -> w475
            frame False {
            }
            frame True {
              n366 = local read "xyhc_out"() -> (w533:T3)
              n367 = Unbundle By Name(w533) -> ("idx"=w498:i32)
              n368 = local read "path_updated"() -> (w532:dbl[][])
              n369 = Add(x=w498, y=w497) -> (x+y=w496:i32)
              n370 = Decrement(x=w496) -> (x-1=w531:i32)
              n371 = Index Array(array=w532, index (col)=w531) -> (element=w530:dbl[])  [unwired: 1 in]
              n372 = Replace Array Subset(array=w530, new element=w499, index=3) -> (w493:dbl[])
              n373 = disable-structure shown="Enabled" {
                disable-tunnel: w493 -> [w535 w548]
                disable-tunnel: [w534 w548] -> w492
                frame Disabled {
                  n374 = flat-sequence {
                    tunnel: w535 -> [w545]
                    tunnel: [w544] -> w534
                    frame #0 {
                      n375 = Index Array(array=w545, index #1=0 ("index"), index #2=1 ("index")) -> (element #1=w542:dbl, element #2=w539:dbl)
                      n376 = global read "G_PATH.vi" "xt"() -> (w547:dbl)
                      n377 = global read "G_PATH.vi" "yt"() -> (w546:dbl)
                      n378 = Add(x=w542, y=w547) -> (x+y=w540:dbl)
                      n379 = Add(x=w539, y=w546) -> (x+y=w538:dbl)
                      n380 = Replace Array Subset(array=w545, new element #1=w540, index #1=0 ("index"), new element #2=w538, index #2=1 ("index")) -> (w544:dbl[])
                    }
                  }
                }
                frame Enabled {
                }
              }
              n381 = Index Array(array=w492, index #1=2 ("index"), index #2=3 ("index"), index #5=3 ("index"), index #6=0 ("index"), index #12=3 ("index")) -> (element #2=w514:dbl, element #3=w515:dbl, element #4=w516:dbl, element #5=w518:dbl, element #6=w521:dbl, element #7=w522:dbl, element #8=w528:dbl, element #9=w523:dbl, element #10=w524:dbl, element #11=w525:dbl, element #12=w527:dbl)  [unwired: 7 in, 1 out]
              n382 = Compound Arithmetic op=MULTIPLY(w514, w514, w514, w515) -> (w512:dbl)
              n383 = Compound Arithmetic op=MULTIPLY(w516, w518, w518) -> (w511:dbl)
              n384 = Compound Arithmetic op=MULTIPLY(3.0 ("value"), w523, w523, w524) -> (w509:dbl)
              n385 = Compound Arithmetic op=MULTIPLY(w525, w527, 2.0 ("value")) -> (w510:dbl)
              n386 = Add(x=w512, y=w511) -> (x+y=w504:dbl)
              n387 = Add(x=w509, y=w510) -> (x+y=w506:dbl)
              n388 = Inverse Tangent(1:w506) -> (0:w505:dbl)
              n389 = call "rotm_siso.vi"("angle[rad]"=w528, "reverse"=TRUE, "y0"=w522, "x0"=w521, "y"=w504, "x"=w514) -> ("y'"=w501:dbl, "x'"=w502:dbl)  [unwired: 4 in]
              n390 = call "headingoperater.vi"("h1"=w505, "h2"=w528) -> ("h2+h1"=w500:dbl)  [unwired: 8 in, 1 out]
              n391 = Bundle By Name(cluster=T2 {"idx"=0, "x"=0.0, "y"=0.0, "hp"=0.0, "x_path"=0.0} ("xyhp"), "idx"=w496, "x"=w502, "y"=w501, "hp"=w500, "x_path"=w499) -> (w495:T2)
            }
          }
        }
        frame True {
        }
      }
      "xyhp" <- w472
    }
  }
